vi "Match First String part 9.vi"() -> ()   [LabVIEW 2020]
panel:
  out "output string":string
  in  "string array":string[](array[string])
  in  "string":string
  # "Match First String"
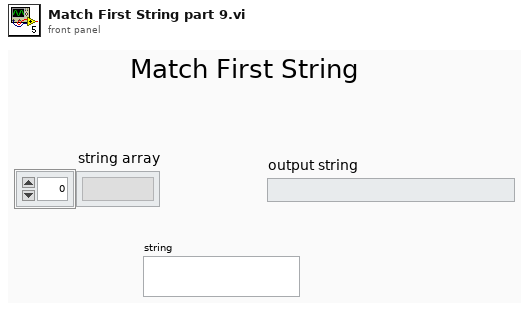
[diagram p1: front panel]
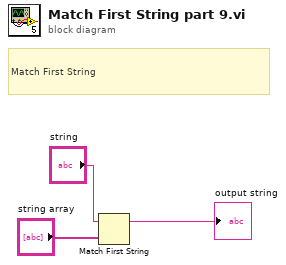
[diagram p0: block diagram]
diagram:
  # "Match First String"
  n1 = Match First String(2:"string array", 3:"string") -> (0:w1:i32, 1:→"output string":string)
